vi "CalcWristFF.vi"(11 "Ticks (from vertical)":dbl) -> (3 "Vert Force Scalar":dbl)   [LabVIEW 2018]
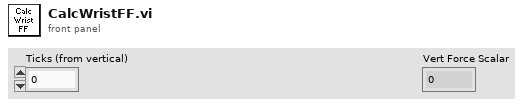
[diagram p1: front panel]
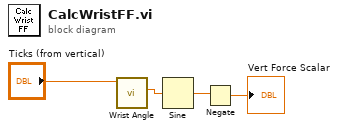
[diagram p0: block diagram]
diagram:
  n1 = call "Wrist Angle.vi"("Ticks (from vertical)"="Ticks (from vertical)") -> ("Angle (Radians)"=w3:dbl)  [unwired: 9 in, 1 out]
  n2 = Sine(x=w3) -> (sin(x)=w2:dbl)
  n3 = Negate(x=w2) -> (-x=→"Vert Force Scalar":dbl)
